vi "TW Updated Default Value for Launch.vi"(8 "error in":errorcluster, 10 "New Subname":string, 11 "Name to VI Map":map{string, refnum<vi>}(c390)) -> (0 "error out":errorcluster)   [LabVIEW 2021, in "Plugin Generator.lvlib"]
uses:
  Plugin Generator.lvlib
  <vilib>/Utility/traverseref.llb/TRef TravTarget.ctl
  <vilib>/Utility/traverseref.llb/VI Scripting - Traverse.lvlib
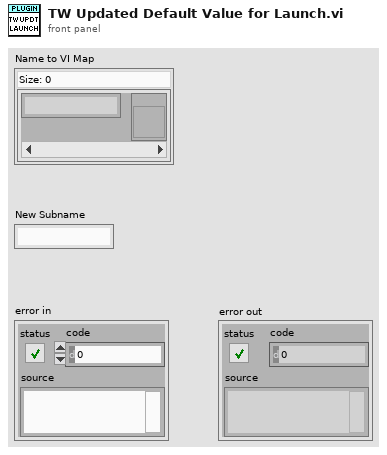
[diagram p1: front panel]
types:
  T1 = typedef "TRef TravTarget.ctl" = enum16{"FP", "BD", "Other"}
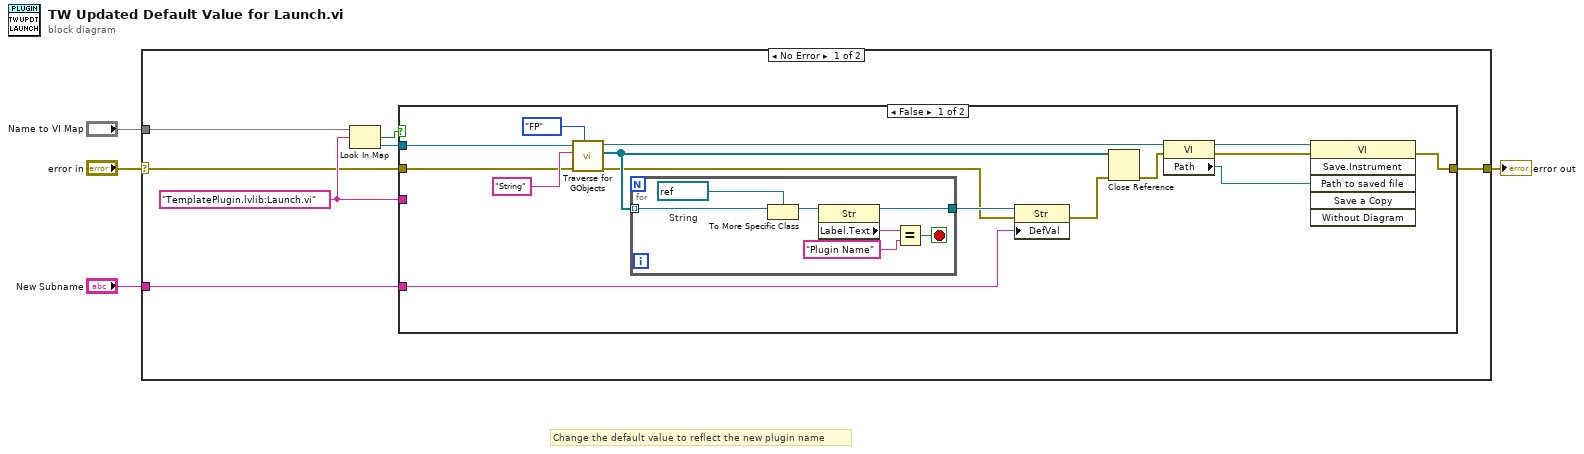
[diagram p0: block diagram]
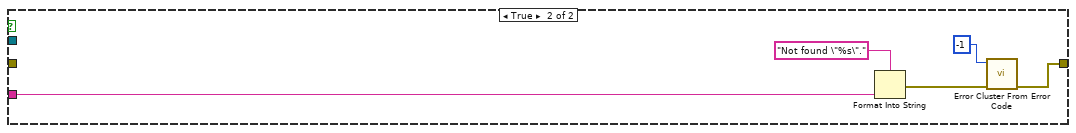
[diagram p2: hidden frame]
diagram:
  # "Change the default value to reflect the new plugin name"
  n1 = case shown="No Error" "error in" {
    selector: "error in" -> [w6 w39]
    tunnel: [w11 w39] -> w4
    tunnel: "New Subname" -> [w10 _]
    tunnel: "Name to VI Map" -> [w5 _]
    frame No Error {
      w8 = "TemplatePlugin.lvlib:Launch.vi" ("String")
      n2 = Look In Map(map=w5, key=w8) -> (key not found?=w7:bool, value=w9:refnum<vi>)  [unwired: 1 in]
      n3 = case shown="False" w7 {
        tunnel: [w14 w38] -> w11
        tunnel: w10 -> [w17 _]
        tunnel: w9 -> [w13 _]
        tunnel: w8 -> [_ w34]
        tunnel: w6 -> [w12 _]
        frame False {
          n4 = call <vilib>:"Traverse for GObjects.vi"("Traverse Target"=TRef_TravTarget."FP", "error in (no error)"=w12, "Class Name"="String", "VI Refnum"=w13) -> ("error out"=w16:errorcluster, "References"=w24:refnum<vi>[], "dup VI Refnum"=w21:refnum<vi>)  [unwired: 4 in, 1 out]
          n5 = for {
            tunnel: w24 -> [w33] mode=indexing
            tunnel: [w28] -> w18
            stop <- w29 stop-if-true
            w32 = refnum<vi> refnum  # String
            n6 = To More Specific Class(target class=w32, reference=w33) -> (specific class reference=w31:refnum<vi>)  [unwired: 1 in, 1 out]
            n7 = property class="Str"(reference=w31) -> (reference out=w28:refnum<vi>, "Label.Text"=w27:string)  [unwired: 1 in, 1 out]
            n8 = Equal?(x=w27, y="Plugin Name") -> (x = y?=w29:bool)
          }
          n9 = property class="Str"(reference=w18, error in=w16, "DefVal"=w17) -> (error out=w15:errorcluster)  [unwired: 1 out]
          n10 = Close Reference(reference=w24, error in (no error)=w15) -> (error out=w20:errorcluster)
          n11 = property class="VI"(reference=w21, error in=w20) -> (reference out=w26:refnum<vi>, error out=w25:errorcluster, "Path"=w19:path)
          n12 = invoke class="VI" method="Save.Instrument"(reference=w26, error in=w25, "Path to saved file"=w19) -> (error out=w14:errorcluster)  [unwired: 3 in, 5 out]
        }
        frame True {
          n13 = Format Into String(format string="Not found \"%s\"." ("error message (\"\")"), w34) -> (error out=w36:errorcluster)  [unwired: 2 in, 1 out]
          n14 = call <vilib>:"Error Cluster From Error Code.vi"("error in (no error)"=w36, "error code (0)"=-1) -> ("error out"=w38:errorcluster)  [unwired: 7 in]
        }
      }
    }
    frame Error {
    }
  }
  "error out" <- w4
